vi "Embedded Server.vi"() -> ()   [LabVIEW 2023]
uses:
  Log/Log_Level.ctl
  API Message/API Message.lvclass
  WebSocket/WebSocket.lvclass
  Log/Log_Facilities.ctl
  Response/Standard Response Messages.ctl
  baea4f90-ed66-40c9-855f-b5689293d002.vi
  baea4f90-ed66-40c9-855f-b5689293d002.vi/bf0030c7-b76b-4182-9f9e-16cd2e366061.vi
  Request/Get Request.vi
  Response/Set Body.vi
  Response/Set Content Type.vi
  Response/Set Status Code.vi
  Response/Send.vi
  Request/Request.lvclass
  Response/Response.lvclass
  Log/Log.lvclass
  Server/Server.lvclass
panel:
  out "Phase":dbl
  out "Frequency":dbl=1.0
  out "Amplitude":dbl=1.0
  out "#Connections":i32
  out "Waveform Chart":dynamicdata(graph)
  in  "stop":bool
  # "From Windows"
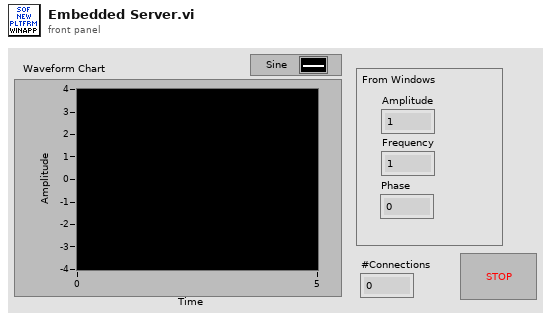
[diagram p1: front panel]
types:
  T1 = typedef "Log.lvclass/Log_Level.ctl" = enum16{"none", "info", "trace", "warn", "error", "fatal"}
  T2 = typedef "Log.lvclass/Log_Facilities.ctl" = string
  T3 = cluster{"type":string, "tag":string, "value":dbl[]}
  T4 = cluster{"type":string, "tag":string, "value":dbl}
  T5 = typedef "Request.ctl" = cluster{"Method":string, "URI":string, "Protocol":string, "Raw Path":string, "Query":string, "Fragment":string, "Raw Body":string, "Headers":variant, "Parameters":variant, "Body":variant, "Raw Header":string, "Path":string[]}
  T6 = typedef "Response.lvclass/Standard Response Messages.ctl" = u16
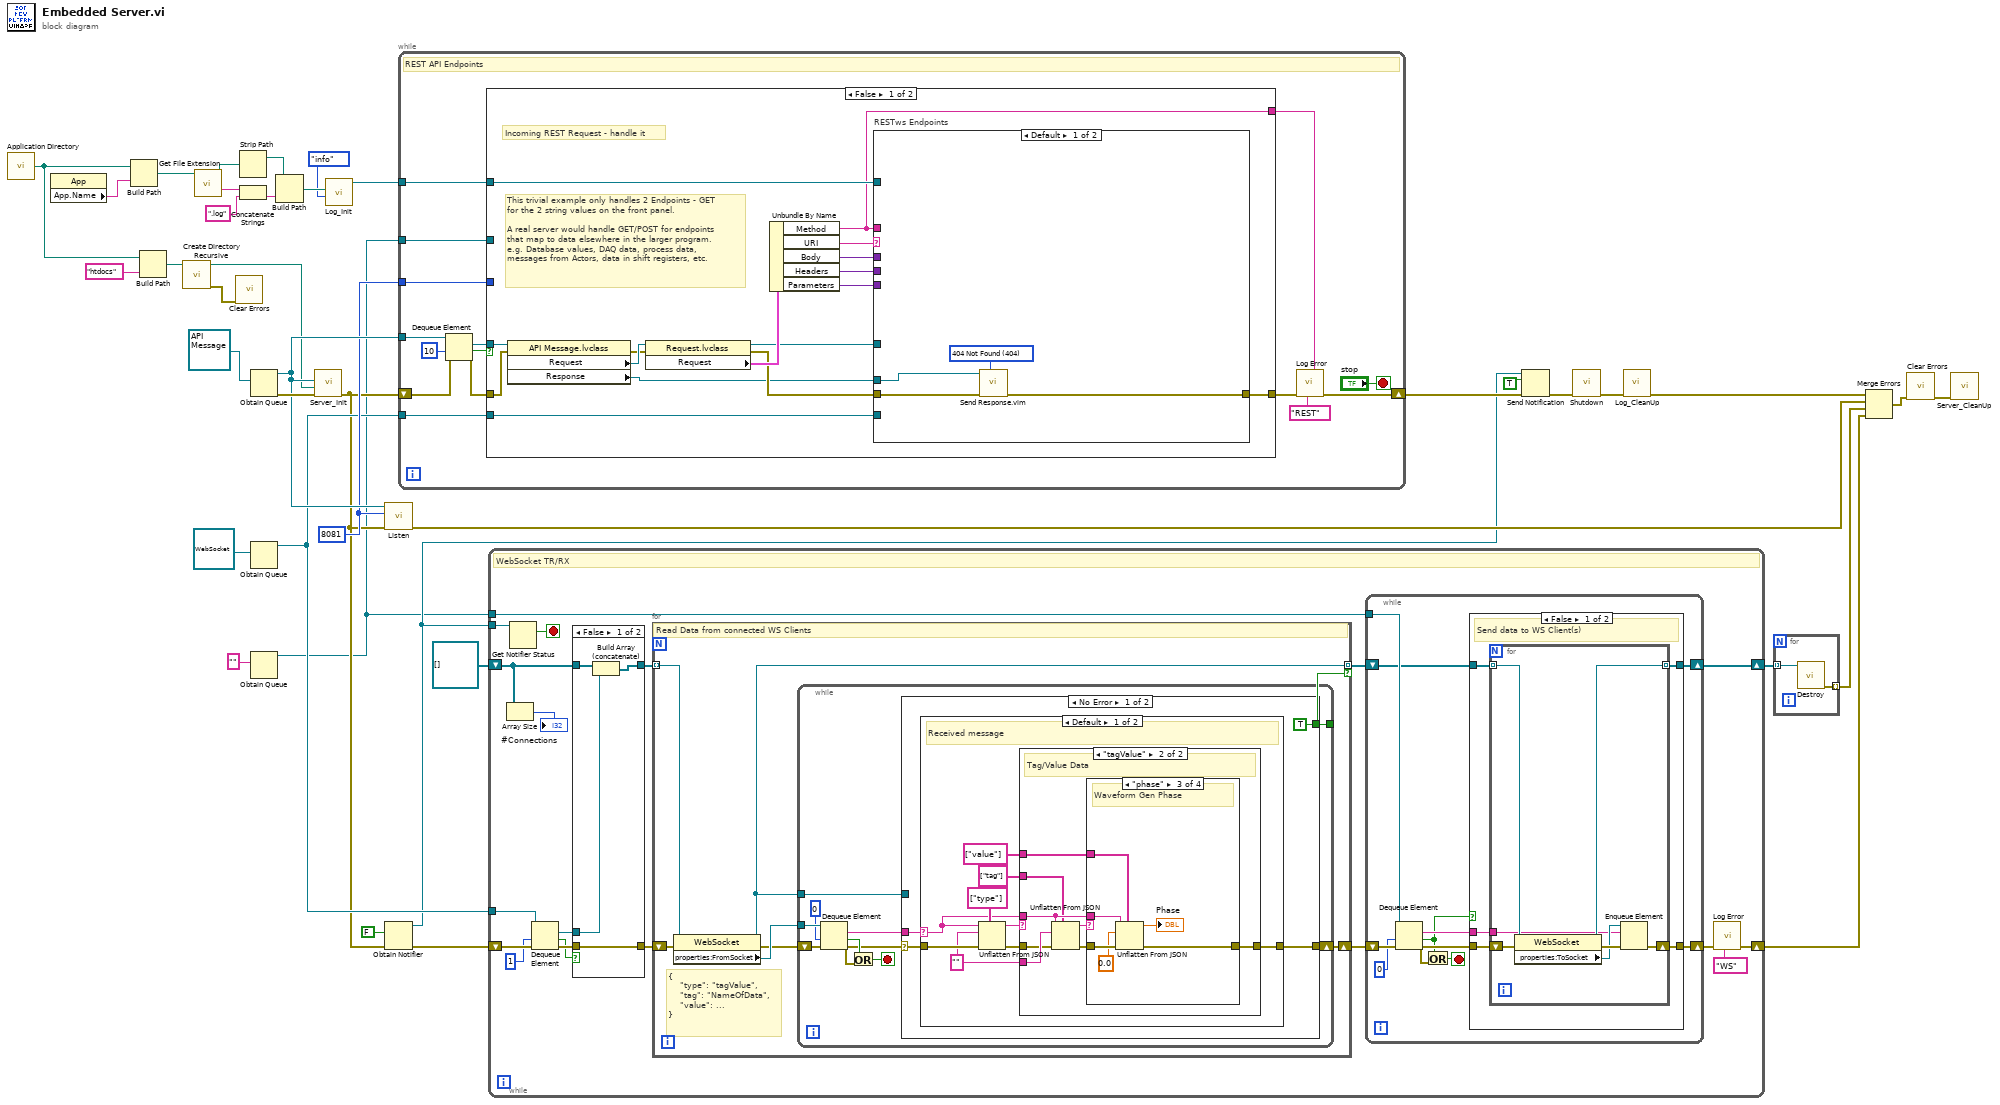
[diagram p0: block diagram]
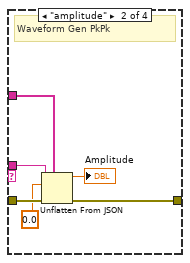
[diagram p5: hidden frame]
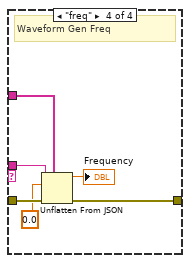
[diagram p6: hidden frame]
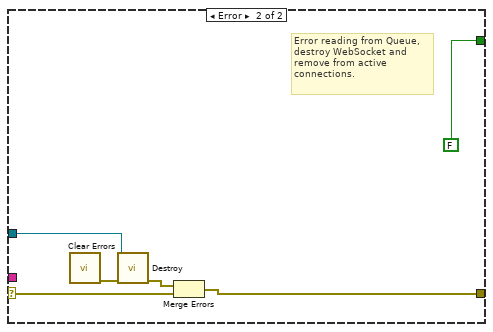
[diagram p8: hidden frame]
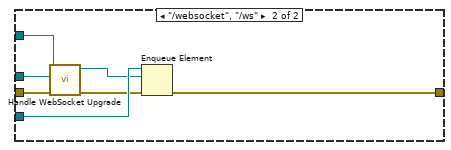
[diagram p10: hidden frame]
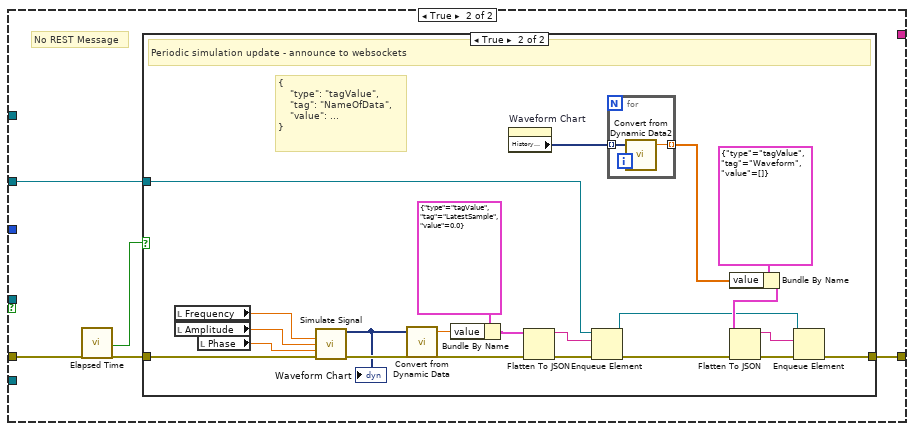
[diagram p11: hidden frame]
diagram:
  w19 = u16 8081 ("Listen Port (80)")
  n1 = call <vilib>:"Application Directory.vi"() -> ("Application Directory"=w30:path)
  n2 = property class="App"() -> ("App.Name"=w26:string)  [unwired: 2 in, 2 out]
  n3 = Build Path(base path=w30, name or relative path=w26) -> (appended path=w27:path)
  n4 = Build Path(base path=w30, name or relative path="htdocs" ("section")) -> (appended path=w18:path)
  n5 = call <vilib>:"Create Directory Recursive.vi"("directory"=w18) -> ("error out"=w16:errorcluster, "directory copy"=w17:path)  [unwired: 4 in, 1 out]
  n6 = call <vilib>:"Get File Extension.vi"("file"=w27) -> ("filename without extension"=w35:string, "dup file"=w34:path)  [unwired: 6 in, 3 out]
  n7 = call <vilib>:"Clear Errors.vi"("error in (no error)"=w16) -> ()  [unwired: 5 in, 2 out]
  n8 = Strip Path(path=w34) -> (stripped path=w33:path)  [unwired: 1 out]
  n9 = Concatenate Strings(w35, ".log" ("section")) -> (w38:string)
  n10 = Obtain Queue(element data type=refnum<class "API Message.lvclass"> refnum ("API Message.lvclass")) -> (queue out=w28:refnum<queue>, error out=w32:errorcluster)  [unwired: 4 in, 1 out]
  n11 = Obtain Queue(element data type=refnum<class "WebSocket.lvclass"> refnum ("WebSocket")) -> (queue out=w14:refnum<queue>)  [unwired: 4 in, 2 out]
  n12 = Obtain Queue(element data type="") -> (queue out=w1:refnum<queue>)  [unwired: 4 in, 2 out]
  n13 = Build Path(base path=w33, name or relative path=w38) -> (appended path=w37:path)
  n14 = call "Server_Init.vi"("error in (no error)"=w32, "Static Data Folder"=w17, "API Queue"=w28) -> ("error out"=w7:errorcluster)  [unwired: 7 in, 1 out]
  n15 = call "Log_Init.vi"("Level"=Log_Level."info", "Log File"=w37) -> ("reference out"=w23:refnum<class "Log.lvclass">)  [unwired: 8 in, 1 out]
  n16 = call "Listen.vi"("error in (no error)"=w7, "Listen Port (80)"=w19, "API Queue"=w28) -> ("error out"=w24:errorcluster)  [unwired: 8 in]
  n17 = Obtain Notifier(notification data type=FALSE, error in (no error)=w7) -> (notifier out=w10:refnum<notifier>, error out=w6:errorcluster)  [unwired: 2 in, 1 out]
  n18 = while "Send to RT" {
    shift-right: [w45] -> w12
    shift-left: w7 -> [w49]
    tunnel: w28 -> [w54]
    tunnel: w23 -> [w47]
    tunnel: w19 -> [w42]
    tunnel: w14 -> [w41]
    tunnel: w1 -> [w40]
    stop <- "stop" stop-if-true
    # "REST API Endpoints"
    n19 = Dequeue Element(queue=w54, timeout in ms (-1)=10, error in (no error)=w49) -> (element=w51:refnum<class "API Message.lvclass">, timed out?=w53:bool, error out=w52:errorcluster)  [unwired: 1 out]
    n20 = case shown="False" w53 {
      tunnel: w52 -> [w69 w86]
      tunnel: [w63 w83] -> w46
      tunnel: w51 -> [w70 _]
      tunnel: w47 -> [w59 _]
      tunnel: [w58 _] -> w43
      tunnel: w42 -> [_ _]
      tunnel: w41 -> [w55 _]
      tunnel: w40 -> [_ w82]
      frame False {
        # "This trivial example only handles 2 Endpoints - GET\nfor the 2 string values on the front panel.\n\nA real server would handle GET/POST for endpoints\nthat map to data elsewhere in the larger program.\ne.g. Database values, DAQ data, process data, \nmessages from Actors, data in shift registers, etc."
        # "Incoming REST Request - handle it"
        n21 = property class="API Message.lvclass"(reference=w70, error in=w69) -> (error out=w67:errorcluster, "Request"=w68:refnum<class "Request.lvclass">, "Response"=w61:refnum<class "Response.lvclass">)  [unwired: 1 out]
        n22 = property class="Request.lvclass"(reference=w68, error in=w67) -> (reference out=w62:refnum<class "Request.lvclass">, error out=w64:errorcluster, "Request"=w66:T5)
        n23 = Unbundle By Name(w66) -> ("Method"=w58:string, "URI"=w65:string, "Body"=w60:variant, "Headers"=w57:variant, "Parameters"=w56:variant)
        n24 = case "RESTws Endpoints" shown="Default" w65 {
          tunnel: w64 -> [w73 w81]
          tunnel: [w74 w76] -> w63
          tunnel: w58 -> [_ _]
          tunnel: w62 -> [_ w80]
          tunnel: w61 -> [w72 w79]
          tunnel: w60 -> [_ _]
          tunnel: w59 -> [_ _]
          tunnel: w57 -> [_ _]
          tunnel: w56 -> [_ _]
          tunnel: w55 -> [_ w78]
          frame Default {
            w71 = T6 404 items=["200 OK"=200, "201 Created"=201, "202 Accepted"=202, "203 Non-Authoritative Information"=203, "204 No Content"=204, "205 Reset Content"=205, "206 Partial Content"=206, "207 Multi-Status (WebDAV)"=207, "208 Already Reported (WebDAV)"=208, "226 IM Used (HTTP Delta encoding)"=226, "300 Multiple Choices"=300, "301 Moved Permanently"=301, "302 Found"=302, "303 See Other"=303, "304 Not Modified"=304, "305 Use Proxy Deprecated"=305, "307 Temporary Redirect"=307, "308 Permanent Redirect"=308, "400 Bad Request"=400, "401 Unauthorized"=401, "402 Payment Required"=402, "403 Forbidden"=403, "404 Not Found"=404, "405 Method Not Allowed"=405, "406 Not Acceptable"=406, "407 Proxy Authentication Required"=407, "408 Request Timeout"=408, "409 Conflict"=409, "410 Gone"=410, "411 Length Required"=411, "412 Precondition Failed"=412, "413 Content Too Large"=413, "414 URI Too Long"=414, "415 Unsupported Media Type"=415, "416 Range Not Satisfiable"=416, "417 Expectation Failed"=417, "418 I'm a teapot"=418, "421 Misdirected Request"=421, "422 Unprocessable Content (WebDAV)"=422, "423 Locked (WebDAV)"=423, "424 Failed Dependency (WebDAV)"=424, "425 Too Early Experimental"=425, "426 Upgrade Required"=426, "428 Precondition Required"=428, "429 Too Many Requests"=429, "431 Request Header Fields Too Large"=431, "451 Unavailable For Legal Reasons"=451, "500 Internal Server Error"=500, "501 Not Implemented"=501, "502 Bad Gateway"=502, "503 Service Unavailable"=503, "504 Gateway Timeout"=504, "505 HTTP Version Not Supported"=505, "506 Variant Also Negotiates"=506, "507 Insufficient Storage (WebDAV)"=507, "508 Loop Detected (WebDAV)"=508, "510 Not Extended"=510, "511 Network Authentication Required"=511] ("Status Codes")
            n25 = call "Send Response.vim"("Status Code (200=OK)"=w71, "Error In"=w73, "Response"=w72) -> ("Error Out"=w74:errorcluster)  [unwired: 8 in]
          }
          frame "/websocket", "/ws" {
            n26 = call "Handle WebSocket Upgrade.vi"("error in (no error)"=w81, "Response.lvclass"=w79, "Request.lvclass"=w80) -> ("error out"=w77:errorcluster, "WebSocket"=w75:refnum<class "WebSocket.lvclass">)  [unwired: 7 in]
            n27 = Enqueue Element(queue=w78, element=w75, error in (no error)=w77) -> (error out=w76:errorcluster)  [unwired: 1 in, 2 out]
          }
        }
      }
      frame True {
        # "No REST Message"
        n28 = call "Elapsed Time"("error in (no error)"=w86) -> ("Time has Elapsed"=w85:bool, "error out"=w84:errorcluster)  [unwired: 11 in, 6 out]
        n29 = case shown="True" w85 {
          tunnel: w84 -> [w87 w107]
          tunnel: [w87 w95] -> w83
          tunnel: w82 -> [_ w94]
          frame False {
          }
          frame True {
            # "{\n    \"type\": \"tagValue\",\n    \"tag\": \"NameOfData\",\n    \"value\": ...\n}"
            # "Periodic simulation update - announce to websockets"
            n30 = local read "Frequency"() -> (w92:dbl)
            n31 = local read "Amplitude"() -> (w91:dbl)
            n32 = local read "Phase"() -> (w90:dbl)
            n33 = call "Simulate Signal"("Frequency"=w92, "Amplitude"=w91, "Phase"=w90, "error in (no error)"=w107) -> ("Sine"=w106:dynamicdata, "error out"=w108:errorcluster)  [unwired: 10 in]
            "Waveform Chart" <- w106
            n34 = call "Convert from Dynamic Data"("Dynamic Data Type"=w106) -> ("Scalar"=w104:dbl)  [unwired: 3 in]
            n35 = Bundle By Name(cluster=T4 {"type"="tagValue", "tag"="LatestSample", "value"=0.0}, "value"=w104) -> (w100:T4)
            n36 = property on="Waveform Chart" class="WFChart (strict)"() -> ("History Data"=w89:dynamicdata[])  [unwired: 2 in, 2 out]
            n37 = Flatten To JSON(anything=w100, error in (no error)=w108) -> (JSON string=w99:string, 11:w101:errorcluster)  [unwired: 1 in]
            n38 = Enqueue Element(queue=w94, element=w99, error in (no error)=w101) -> (queue out=w93:refnum<queue>, error out=w102:errorcluster)  [unwired: 1 in, 1 out]
            n39 = for {
              tunnel: w89 -> [w110] mode=indexing
              tunnel: [w109] -> w88 mode=indexing
              n40 = call "Convert from Dynamic Data2"("Dynamic Data Type"=w110) -> ("Scalar"=w109:dbl)  [unwired: 3 in]
            }
            n41 = Bundle By Name(cluster=T3 {"type"="tagValue", "tag"="Waveform", "value"=[]}, "value"=w88) -> (w98:T3)
            n42 = Flatten To JSON(anything=w98, error in (no error)=w102) -> (JSON string=w97:string, 11:w96:errorcluster)  [unwired: 1 in]
            n43 = Enqueue Element(queue=w93, element=w97, error in (no error)=w96) -> (error out=w95:errorcluster)  [unwired: 1 in, 2 out]
          }
        }
      }
    }
    n44 = call "Log Error.vi"("Context"=w43, "Facility (default)"=T2 "REST", "error in (no error)"=w46) -> ("error out"=w45:errorcluster)  [unwired: 8 in]
  }
  n45 = while {
    tunnel: w14 -> [w122]
    shift-right: [w119] -> w3
    shift-left: w6 -> [w129]
    shift-right: [w114] -> w5
    shift-left: refnum<class "WebSocket.lvclass">[] [] -> [w112]
    tunnel: w10 -> [w124]
    tunnel: w1 -> [w121]
    stop <- w123 stop-if-true
    # "WebSocket TR/RX"
    n46 = Array Size(array=w112) -> (size(s)=→"#Connections":i32)
    n47 = Get Notifier Status(notifier=w124) -> (current notification=w123:bool)  [unwired: 1 in, 4 out]
    n48 = Dequeue Element(queue=w122, timeout in ms (-1)=1, error in (no error)=w129) -> (element=w125:refnum<class "WebSocket.lvclass">, timed out?=w126:bool, error out=w127:errorcluster)  [unwired: 1 out]
    n49 = case shown="False" w126 {
      tunnel: w127 -> [w219 w223]
      tunnel: w125 -> [w222 _]
      tunnel: w112 -> [w221 w224]
      tunnel: [w220 w224] -> w118
      tunnel: [w219 w223] -> w117
      frame False {
        n50 = Build Array (concatenate)(w221, w222) -> (w220:refnum<class "WebSocket.lvclass">[])
      }
      frame True {
      }
    }
    n51 = for {
      tunnel: w118 -> [w159] mode=indexing
      shift-right: [w156] -> w116
      shift-left: w117 -> [w160]
      tunnel: [w154] -> w115 mode=indexing if=w155
      # "{\n    \"type\": \"tagValue\",\n    \"tag\": \"NameOfData\",\n    \"value\": ...\n}"
      # "Read Data from connected WS Clients"
      n52 = property class="WebSocket"(reference=w159, error in=w160) -> (reference out=w154:refnum<class "WebSocket.lvclass">, error out=w157:errorcluster, "properties:FromSocket"=w158:refnum<queue>)
      n53 = while {
        tunnel: w158 -> [w170]
        tunnel: [w165] -> w155
        tunnel: w154 -> [w164]
        shift-right: [w166] -> w156
        shift-left: w157 -> [w168]
        stop <- w161 stop-if-true
        n54 = Dequeue Element(queue=w170, timeout in ms (-1)=0, error in (no error)=w168) -> (element=w167:string, timed out?=w163:bool, error out=w162:errorcluster)  [unwired: 1 out]
        n55 = Or(x=w163, y=w162) -> (x .or. y?=w161:bool)
        n56 = case shown="No Error" w162 {
          selector: w162 -> [w172 w217]
          tunnel: w167 -> [w173 _]
          tunnel: [w171 w213] -> w166
          tunnel: [TRUE FALSE] -> w165
          tunnel: w164 -> [_ w215]
          frame No Error {
            n57 = case shown="Default" w173 {
              selector: w173 -> [w178 _]
              tunnel: w172 -> [w183 w212]
              tunnel: [w179 w212] -> w171
              frame Default {
                w177 = ""
                # "Received message"
                n58 = Unflatten From JSON(path=string[] ["type"], JSON string=w178, type and defaults=w177, error in (no error)=w183) -> (value=w180:string, error out=w181:errorcluster)  [unwired: 3 in]
                n59 = case shown="\"tagValue\"" w180 {
                  tunnel: w181 -> [w184 w191]
                  tunnel: [w184 w190] -> w179
                  tunnel: w178 -> [_ w187]
                  tunnel: w177 -> [_ w192]
                  tunnel: string[] ["tag"] -> [_ w186]
                  tunnel: string[] ["value"] -> [_ w185]
                  frame Default {
                    # "Unknown Packet Type"
                  }
                  frame "tagValue" {
                    # "Tag/Value Data"
                    n60 = Unflatten From JSON(path=w186, JSON string=w187, type and defaults=w192, error in (no error)=w191) -> (value=w188:string, error out=w189:errorcluster)  [unwired: 3 in]
                    n61 = case shown="\"phase\"" w188 {
                      tunnel: [w193 w198 w204 w210] -> w190
                      tunnel: w189 -> [w193 w199 w205 w211]
                      tunnel: w187 -> [_ w197 w203 w209]
                      tunnel: w185 -> [_ w195 w201 w207]
                      frame Default {
                        # "Unknown Tag"
                      }
                      frame "amplitude" {
                        # "Waveform Gen PkPk"
                        n62 = Unflatten From JSON(path=w195, JSON string=w197, type and defaults=0.0, error in (no error)=w199) -> (value=→"Amplitude":dbl, error out=w198:errorcluster)  [unwired: 3 in]
                      }
                      frame "phase" {
                        # "Waveform Gen Phase"
                        n63 = Unflatten From JSON(path=w201, JSON string=w203, type and defaults=0.0, error in (no error)=w205) -> (value=→"Phase":dbl, error out=w204:errorcluster)  [unwired: 3 in]
                      }
                      frame "freq" {
                        # "Waveform Gen Freq"
                        n64 = Unflatten From JSON(path=w207, JSON string=w209, type and defaults=0.0, error in (no error)=w211) -> (value=→"Frequency":dbl, error out=w210:errorcluster)  [unwired: 3 in]
                      }
                    }
                  }
                }
              }
              frame "" {
              }
            }
          }
          frame Error {
            # "Error reading from Queue,\ndestroy WebSocket and\nremove from active\nconnections."
            n65 = call <vilib>:"Clear Errors.vi"() -> ("error out"=w216:errorcluster)  [unwired: 6 in, 1 out]
            n66 = call-dynamic "Destroy.vi"("error in (no error)"=w216, "reference in"=w215) -> ("error out"=w214:errorcluster)  [unwired: 8 in, 1 out]
            n67 = Merge Errors(w214, w217) -> (w213:errorcluster)
          }
        }
      }
    }
    n68 = while {
      tunnel: w121 -> [w139]
      shift-right: [w134] -> w113
      shift-left: w116 -> [w137]
      shift-right: [w135] -> w114
      shift-left: w115 -> [w136]
      stop <- w130 stop-if-true
      n69 = Dequeue Element(queue=w139, timeout in ms (-1)=0, error in (no error)=w137) -> (element=w138:string, timed out?=w131:bool, error out=w132:errorcluster)  [unwired: 1 out]
      n70 = Or(x=w131, y=w132) -> (x .or. y?=w130:bool)
      n71 = case shown="False" w131 {
        tunnel: w132 -> [w144 w153]
        tunnel: w138 -> [w143 _]
        tunnel: w136 -> [w142 w152]
        tunnel: [w141 w152] -> w135
        tunnel: [w140 w153] -> w134
        frame False {
          # "Send data to WS Client(s)"
          n72 = for {
            shift-right: [w146] -> w140
            shift-left: w144 -> [w151]
            tunnel: w143 -> [w145]
            tunnel: w142 -> [w150] mode=indexing
            tunnel: [w147] -> w141 mode=indexing
            n73 = property class="WebSocket"(reference=w150, error in=w151) -> (reference out=w147:refnum<class "WebSocket.lvclass">, error out=w149:errorcluster, "properties:ToSocket"=w148:refnum<queue>)
            n74 = Enqueue Element(queue=w148, element=w145, error in (no error)=w149) -> (error out=w146:errorcluster)  [unwired: 1 in, 2 out]
          }
        }
        frame True {
        }
      }
    }
    n75 = call "Log Error.vi"("Facility (default)"=T2 "WS", "error in (no error)"=w113) -> ("error out"=w119:errorcluster)  [unwired: 9 in]
  }
  n76 = Send Notification(notification=TRUE, notifier=w10, error in (no error)=w12) -> (error out=w11:errorcluster)  [unwired: 1 out]
  n77 = call "Shutdown.vi"("error in (no error)"=w11) -> ("error out"=w21:errorcluster)  [unwired: 10 in]
  n78 = call "Log_CleanUp.vi"("error in (no error)"=w21) -> ("error out"=w22:errorcluster)  [unwired: 10 in]
  n79 = for {
    tunnel: w5 -> [w226] mode=indexing
    tunnel: [w225] -> w4 mode=indexing
    n80 = call-dynamic "Destroy.vi"("reference in"=w226) -> ("error out"=w225:errorcluster)  [unwired: 9 in, 1 out]
  }
  n81 = Merge Errors(w22, w24, w4, w3) -> (w25:errorcluster)
  n82 = call <vilib>:"Clear Errors.vi"("error in (no error)"=w25) -> ("error out"=w20:errorcluster)  [unwired: 5 in, 1 out]
  n83 = call "Server_CleanUp.vi"("error in (no error)"=w20) -> ()  [unwired: 10 in, 1 out]
